vi "tag components to unique name.vi"(10 "Tag Name":string, 11 "Network Path":string) -> (3 "unique name":string)   [LabVIEW 2013, in "EIP Tags Configuration.lvclass"]
uses:
  EIP Tags Configuration.lvclass
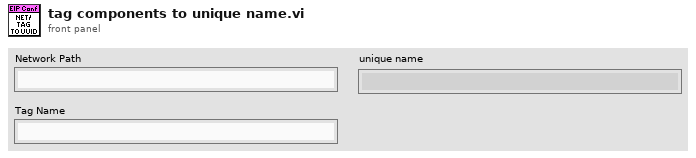
[diagram p1: front panel]
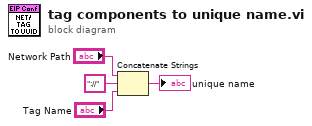
[diagram p0: block diagram]
diagram:
  n1 = Concatenate Strings("Network Path", "://" ("string"), "Tag Name") -> (→"unique name":string)
